vi "tokens_to_expression.vi"(11 "Tokens in":string[](array[string])) -> (2 "Tokens out":string[](array[string]), 3 "Expression out":T1)   [LabVIEW 2020]
uses:
  ExpressionType.ctl
  Expression.ctl
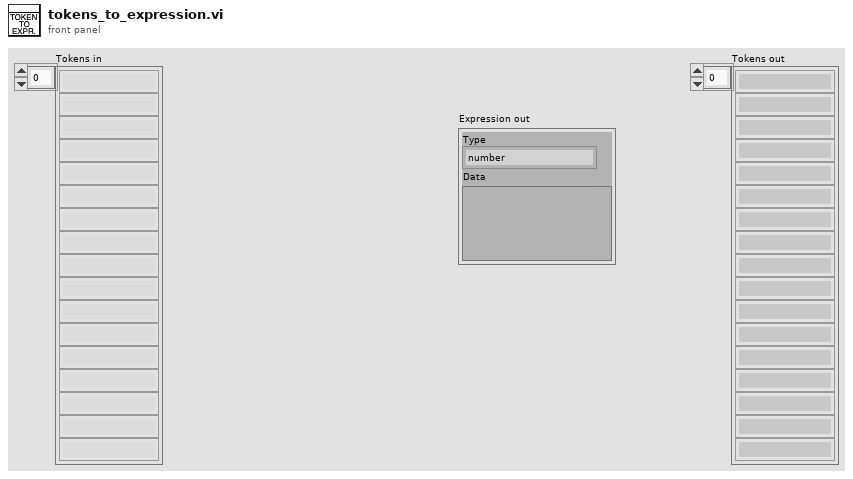
[diagram p1: front panel]
types:
  T1 = typedef "Expression.ctl" = cluster{"Type":T2, "Data":variant}
  T2 = typedef "ExpressionType.ctl" = enum16{"number", "string", "symbol", "primitive", "list", "closure", "macro", "nil", "error"}
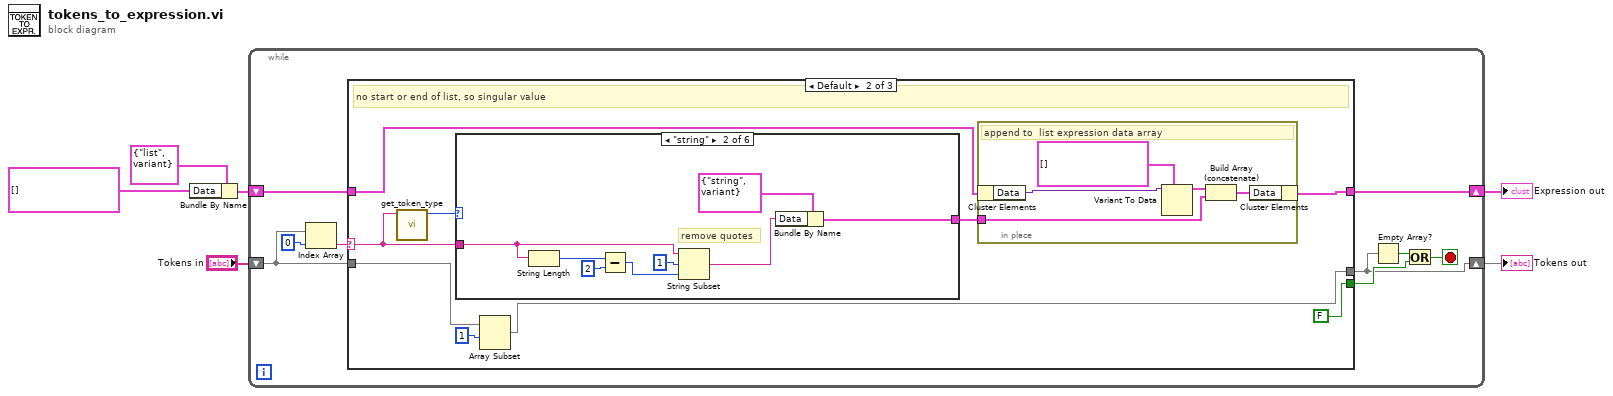
[diagram p0: block diagram]
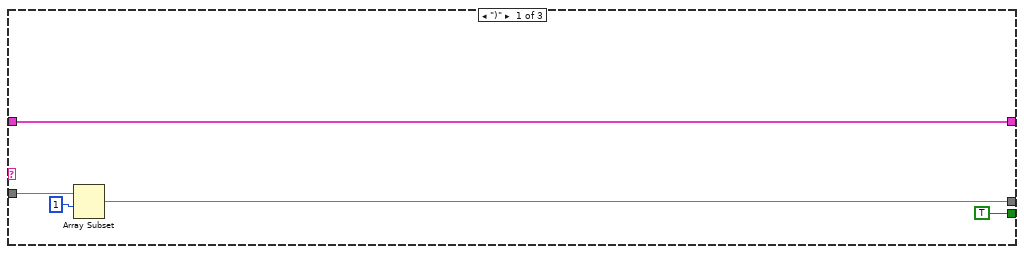
[diagram p2: hidden frame]
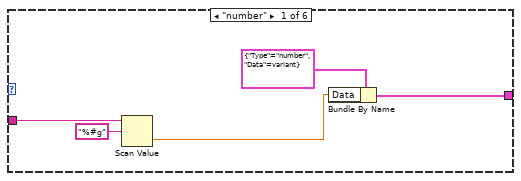
[diagram p3: hidden frame]
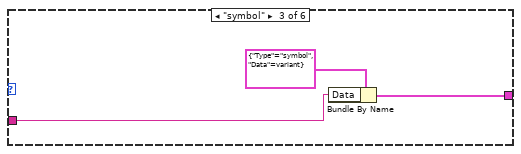
[diagram p4: hidden frame]
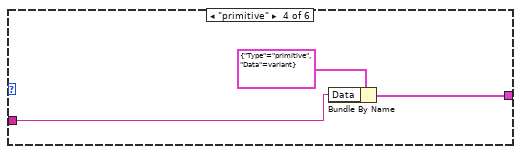
[diagram p5: hidden frame]
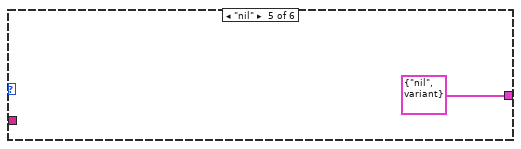
[diagram p6: hidden frame]
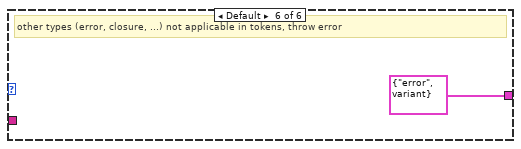
[diagram p7: hidden frame]
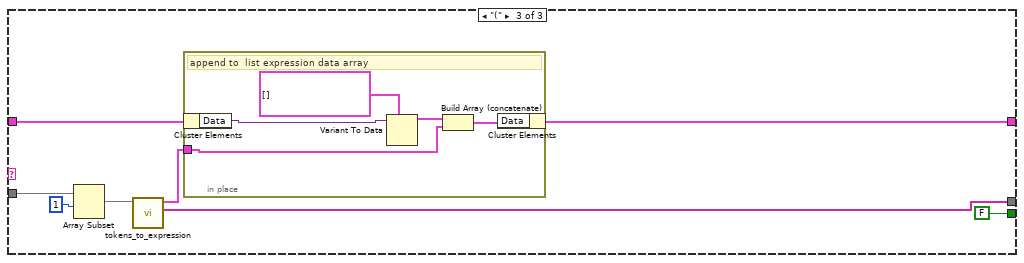
[diagram p8: hidden frame]
diagram:
  n1 = Bundle By Name(cluster=T1 {"Type"=enum."list", "Data"=variant} ("Expression out"), "Data"=T1[] []) -> (w1:T1)
  n2 = while {
    shift-right: [w13] -> w5
    shift-left: w1 -> [w12]
    shift-right: [w7] -> w4
    shift-left: "Tokens in" -> [w11]
    stop <- w10 stop-if-true
    n3 = Index Array(array=w11, index=0) -> (element=w15:string)
    n4 = case shown="Default" w15 {
      selector: w15 -> [_ w27 _]
      tunnel: [TRUE FALSE FALSE] -> w9
      tunnel: [w19 w26 w62] -> w13
      tunnel: w12 -> [w19 w25 w61]
      tunnel: w11 -> [w17 w22 w57]
      tunnel: [w16 w21 w59] -> w7
      frame ")" {
        n5 = Array Subset(array=w17, index=1) -> (w16:string[])  [unwired: 1 in]
      }
      frame Default {
        # "no start or end of list, so singular value"
        n6 = call "get_token_type.vi"("token"=w27) -> ("ExpressionType"=w28:T2)  [unwired: 10 in]
        n7 = case shown="\"string\"" w28 {
          tunnel: w27 -> [w36 w44 w49 w52 _ _]
          tunnel: [w38 w46 w48 w51 T1 {"Type"=enum."nil", "Data"=variant} ("Expression out") T1 {"Type"=enum."error", "Data"=variant} ("Expression out")] -> w24
          frame "number" {
            n8 = Scan Value(string=w36, format string="%#g") -> (value=w35:dbl)  [unwired: 1 in, 1 out]
            n9 = Bundle By Name(cluster=T1 {"Type"=enum."number", "Data"=variant} ("Expression out"), "Data"=w35) -> (w38:T1)
          }
          frame "string" {
            # "remove quotes"
            n10 = String Length(string=w44) -> (length=w43:i32)
            n11 = Subtract(x=w43, y=2) -> (x-y=w42:i32)
            n12 = String Subset(string=w44, offset (0)=1, length (rest)=w42) -> (substring=w40:string)
            n13 = Bundle By Name(cluster=T1 {"Type"=enum."string", "Data"=variant} ("Expression out"), "Data"=w40) -> (w46:T1)
          }
          frame "symbol" {
            n14 = Bundle By Name(cluster=T1 {"Type"=enum."symbol", "Data"=variant} ("Expression out"), "Data"=w49) -> (w48:T1)
          }
          frame "primitive" {
            n15 = Bundle By Name(cluster=T1 {"Type"=enum."primitive", "Data"=variant} ("Expression out"), "Data"=w52) -> (w51:T1)
          }
          frame "nil" {
          }
          frame Default {
            # "other types (error, closure, ...) not applicable in tokens, throw error"
          }
        }
        n16 = Array Subset(array=w22, index=1) -> (w21:string[])  [unwired: 1 in]
        n17 = in-place {
          in-place-border: w24 -> [w30]
          # "append to  list expression data array"
          n18 = in-place-cluster #1(w25) -> ("Data"=w34:variant)
          n19 = Variant To Data(type=T1[] [], Variant=w34) -> (data=w32:T1[])  [unwired: 1 in, 1 out]
          n20 = Build Array (concatenate)(w32, w30) -> (w31:T1[])
          n21 = in-place-cluster #1("Data"=w31) -> (w26:T1)
        }
      }
      frame "(" {
        n22 = Array Subset(array=w57, index=1) -> (w56:string[])  [unwired: 1 in]
        n23 = call "tokens_to_expression.vi"("Tokens in"=w56) -> ("Tokens out"=w59:string[], "Expression out"=w60:T1)  [unwired: 9 in]
        n24 = in-place {
          in-place-border: w60 -> [w64]
          # "append to  list expression data array"
          n25 = in-place-cluster #2(w61) -> ("Data"=w68:variant)
          n26 = Variant To Data(type=T1[] [], Variant=w68) -> (data=w66:T1[])  [unwired: 1 in, 1 out]
          n27 = Build Array (concatenate)(w66, w64) -> (w65:T1[])
          n28 = in-place-cluster #2("Data"=w65) -> (w62:T1)
        }
      }
    }
    n29 = Empty Array?(array=w7) -> (empty?=w8:bool)
    n30 = Or(x=w8, y=w9) -> (x .or. y?=w10:bool)
  }
  "Expression out" <- w5
  "Tokens out" <- w4
